vi "running avg.vi"(11 "Single Encoder Counts Out":i32) -> ()   [LabVIEW 2023, in "Tube Wheel_ACT.lvlib"]
uses:
  Tube Wheel_ACT.lvlib
panel:
  in  "Avg Size":i32=10
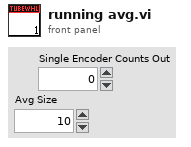
[diagram p1: front panel]
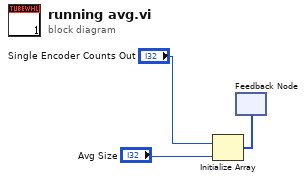
[diagram p0: block diagram]
diagram:
  n1 = Initialize Array("Single Encoder Counts Out", "Avg Size") -> (w3:i32[])
  n2 = feedback #1(w3) -> ()  [unwired: 1 in]
  n3 = feedback-in #1() -> ()  [unwired: 1 out]
